vi "closeDevice.vi"(8 "error in (no error)":errorcluster, 10 "deviceName":string, 11 "BECHWCBasic in":refnum<class "BECHWCBasic.lvclass">) -> (0 "error out":errorcluster, 3 "BECHWCBasic out":refnum<class "BECHWCBasic.lvclass">)   [LabVIEW 2009, in "Hardware.lvlib" / "HWControllers.lvlib" / "BECHWCBasic.lvclass"]
doc: "Shut down a device, so it is no longer in use by labview."
uses:
  BECHWCBasic.lvclass
  BECHWCBasic.lvclass/BECHWCBasic.ctl
  Channels/Digital/DigitalOutput.lvclass
  Channels/VoltOutput/AnalogOutput.lvclass
  IntegrationManagement/CameraManager.lvclass
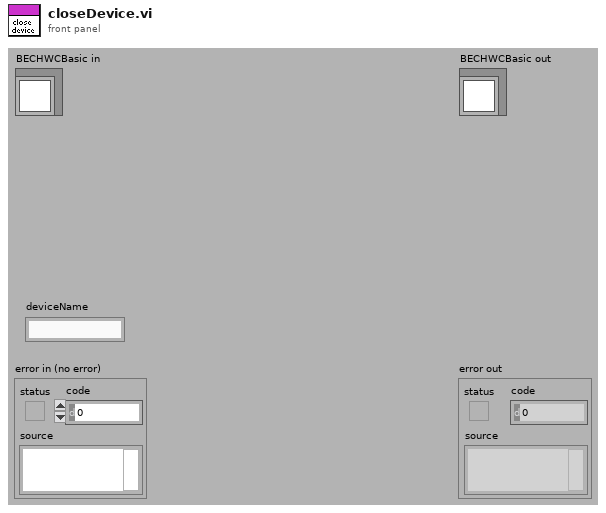
[diagram p1: front panel]
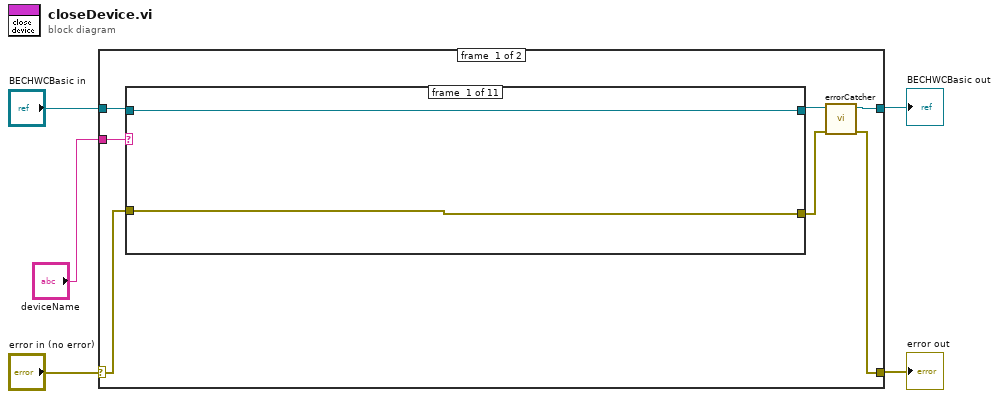
[diagram p0: block diagram]
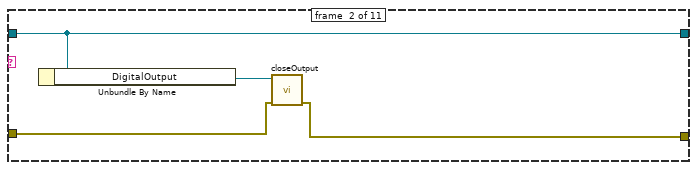
[diagram p2: hidden frame]
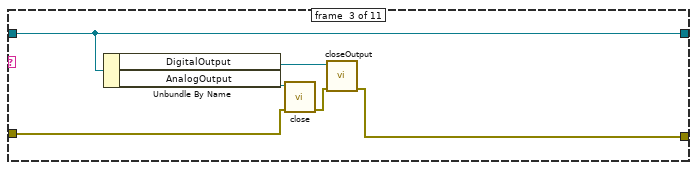
[diagram p3: hidden frame]
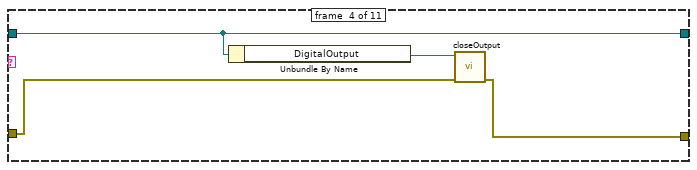
[diagram p4: hidden frame]
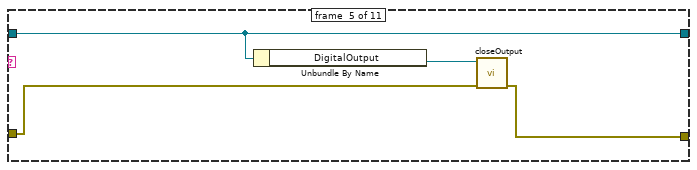
[diagram p5: hidden frame]
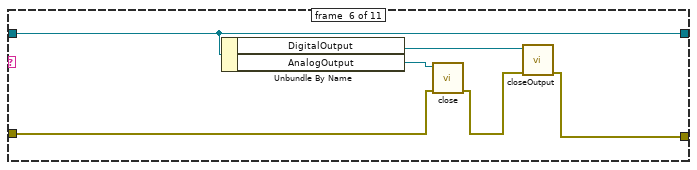
[diagram p6: hidden frame]
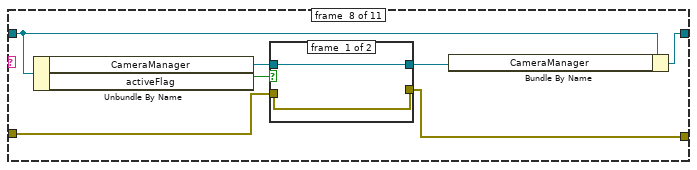
[diagram p8: hidden frame]
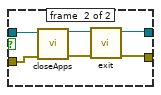
[diagram p9: hidden frame]
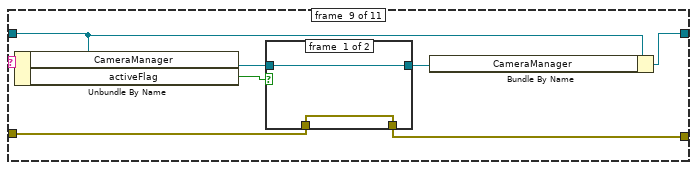
[diagram p10: hidden frame]
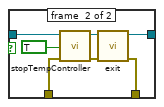
[diagram p11: hidden frame]
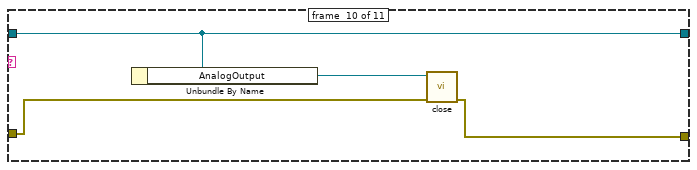
[diagram p12: hidden frame]
diagram:
  n1 = case shown="No Error" "error in (no error)" {
    selector: "error in (no error)" -> [w11 w79]
    tunnel: [w8 w79] -> w4
    tunnel: [w6 w78] -> w2
    tunnel: "BECHWCBasic in" -> [w12 w78]
    tunnel: "deviceName" -> [w10 _]
    frame #0 {
      n2 = case shown="\"Daq\"" w10 {
        tunnel: w12 -> [w14 w18 w23 w27 w31 w37 w40 w44 w58 w75 w77]
        tunnel: [w14 w18 w23 w27 w31 w37 w40 w47 w62 w75 w77] -> w7
        tunnel: w11 -> [w13 w16 w20 w26 w30 w34 w39 w42 w59 w73 w76]
        tunnel: [w13 w15 w22 w25 w29 w36 w39 w45 w60 w72 w76] -> w9
        frame #0 {
        }
        frame #1 {
          n3 = Unbundle By Name(w18) -> ("DigitalOutput"=w17:refnum<class "DigitalOutput.lvclass">)
          n4 = call-dynamic "closeOutput.vi"("error in (no error)"=w16, "DigitalOutput in"=w17) -> ("error out"=w15:errorcluster)  [unwired: 9 in]
        }
        frame #2 {
          n5 = Unbundle By Name(w23) -> ("DigitalOutput"=w24:refnum<class "DigitalOutput.lvclass">, "AnalogOutput"=w21:refnum<class "AnalogOutput.lvclass">)
          n6 = call-dynamic "close.vi"("error in (no error)"=w20, "AnalogOutput in"=w21) -> ("error out"=w19:errorcluster)  [unwired: 9 in]
          n7 = call-dynamic "closeOutput.vi"("error in (no error)"=w19, "DigitalOutput in"=w24) -> ("error out"=w22:errorcluster)  [unwired: 9 in]
        }
        frame #3 {
          n8 = Unbundle By Name(w27) -> ("DigitalOutput"=w28:refnum<class "DigitalOutput.lvclass">)
          n9 = call-dynamic "closeOutput.vi"("error in (no error)"=w26, "DigitalOutput in"=w28) -> ("error out"=w25:errorcluster)  [unwired: 9 in]
        }
        frame #4 {
          n10 = Unbundle By Name(w31) -> ("DigitalOutput"=w32:refnum<class "DigitalOutput.lvclass">)
          n11 = call-dynamic "closeOutput.vi"("error in (no error)"=w30, "DigitalOutput in"=w32) -> ("error out"=w29:errorcluster)  [unwired: 9 in]
        }
        frame #5 {
          n12 = Unbundle By Name(w37) -> ("DigitalOutput"=w38:refnum<class "DigitalOutput.lvclass">, "AnalogOutput"=w35:refnum<class "AnalogOutput.lvclass">)
          n13 = call-dynamic "close.vi"("error in (no error)"=w34, "AnalogOutput in"=w35) -> ("error out"=w33:errorcluster)  [unwired: 9 in]
          n14 = call-dynamic "closeOutput.vi"("error in (no error)"=w33, "DigitalOutput in"=w38) -> ("error out"=w36:errorcluster)  [unwired: 9 in]
        }
        frame #6 {
        }
        frame #7 {
          n15 = Unbundle By Name(w44) -> ("CameraManager"=w43:refnum<class "CameraManager.lvclass">, "activeFlag"=w41:bool)
          n16 = case shown="True" w41 {
            tunnel: [w49 w55] -> w46
            tunnel: [w48 w54] -> w45
            tunnel: w43 -> [w49 w51]
            tunnel: w42 -> [w48 w50]
            frame #0 {
            }
            frame #1 {
              n17 = call "closeApps.vi"("error in (no error)"=w50, "CameraManager in"=w51) -> ("error out"=w53:errorcluster, "CameraManager out"=w52:refnum<class "CameraManager.lvclass">)  [unwired: 8 in]
              n18 = call-dynamic "exit.vi"("error in (no error)"=w53, "CameraManager in"=w52) -> ("error out"=w54:errorcluster, "CameraManager out"=w55:refnum<class "CameraManager.lvclass">)  [unwired: 8 in]
            }
          }
          n19 = Bundle By Name(cluster=w44, "CameraManager"=w46) -> (w47:refnum<class "BECHWCBasic.lvclass">)
        }
        frame #8 {
          n20 = Unbundle By Name(w58) -> ("CameraManager"=w57:refnum<class "CameraManager.lvclass">, "activeFlag"=w56:bool)
          n21 = case shown="True" w56 {
            tunnel: [w64 w70] -> w61
            tunnel: [w63 w65] -> w60
            tunnel: w59 -> [w63 w66]
            tunnel: w57 -> [w64 w67]
            frame #0 {
            }
            frame #1 {
              n22 = call "stopTempController.vi"("error in (no error)"=w66, "releaseWhenReady"=TRUE, "CameraManager in"=w67) -> ("error out"=w69:errorcluster, "CameraManager out"=w68:refnum<class "CameraManager.lvclass">)  [unwired: 7 in]
              n23 = call-dynamic "exit.vi"("error in (no error)"=w69, "CameraManager in"=w68) -> ("error out"=w65:errorcluster, "CameraManager out"=w70:refnum<class "CameraManager.lvclass">)  [unwired: 8 in]
            }
          }
          n24 = Bundle By Name(cluster=w58, "CameraManager"=w61) -> (w62:refnum<class "BECHWCBasic.lvclass">)
        }
        frame #9 {
          n25 = Unbundle By Name(w75) -> ("AnalogOutput"=w74:refnum<class "AnalogOutput.lvclass">)
          n26 = call-dynamic "close.vi"("error in (no error)"=w73, "AnalogOutput in"=w74) -> ("error out"=w72:errorcluster)  [unwired: 9 in]
        }
        frame #10 {
        }
      }
      n27 = call-dynamic "errorCatcher.vi"("error in (no error)"=w9, "HWController in"=w7) -> ("error out"=w8:errorcluster, "HWController out"=w6:refnum<class "BECHWCBasic.lvclass">)  [unwired: 8 in]
    }
    frame #1 {
    }
  }
  "error out" <- w4
  "BECHWCBasic out" <- w2
